vi "FRCts20_Backend_API_Application.vi"(8 "error in (no error)":errorcluster, 10 "Command":T1="Revision") -> (0 "error out":errorcluster, 2 "Status":string, 3 "Application":T2)   [LabVIEW 2014, in "FRCts20_Backend_Engine.lvlib" / "FRCts20_Backend_API.lvlib"]
doc: "This VI could be in charge of controlling the backend, but at present it is not."
uses:
  FRCts20_Backend_API.lvlib
  FRCts20_Backend_API_Application.ctl
  FRCts20_Backend_API_Command_App.ctl
  FRCts20_Backend_FGVOperation.ctl
  FRCts20_Backend_Engine.lvlib
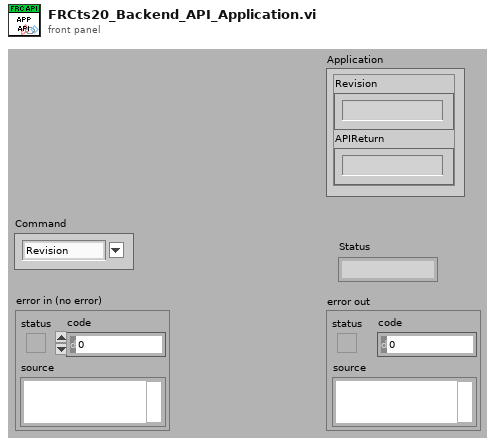
[diagram p1: front panel]
types:
  T1 = typedef "FRCts20_Backend_Engine.lvlib/FRCts20_Backend_API.lvlib/FRCts20_Backend_API_Command_App.ctl" = string
  T2 = typedef "FRCts20_Backend_API_Application.ctl" = cluster{"Revision":string, "APIReturn":string}
  T3 = typedef "FRCts20_Backend_Engine.lvlib/FRCts20_Backend_FGVOperation.ctl" = enum16{"Initialize", "EnqueueMessage", "EnqueueDataReturn", "FlushMessage", "FlushDataReturn"}
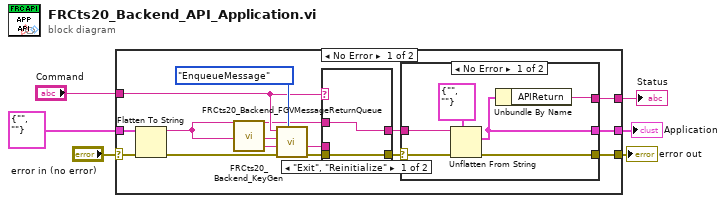
[diagram p0: block diagram]
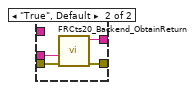
[diagram p2: hidden frame]
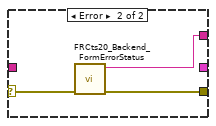
[diagram p3: hidden frame]
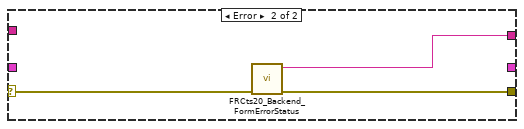
[diagram p4: hidden frame]
diagram:
  n1 = case shown="No Error" "error in (no error)" {
    selector: "error in (no error)" -> [w20 w37]
    tunnel: [w14 w36] -> w5
    tunnel: [w12 w38] -> w4
    tunnel: "Command" -> [w8 _]
    tunnel: [w11 _] -> w2
    tunnel: T2 {"Revision"="", "APIReturn"=""} ("Revision") -> [w10 _]
    frame No Error {
      n2 = Flatten To String(anything=w10, error in (no error)=w20) -> (data string=w7:string, error out=w19:errorcluster)  [unwired: 2 in, 1 out]
      n3 = call "FRCts20_Backend_KeyGen.vi"() -> ("Keygen"=w18:string)  [unwired: 27 in]
      n4 = call "FRCts20_Backend_FGVMessageReturnQueue.vi"("Operation"=FRCts20_Backend_FGVOperation."EnqueueMessage", "error in (no error)"=w19, "Key"=w18, "Message Value"=w7, "Message Name"=w8) -> ("error out"=w16:errorcluster, "Key (Duplicate)"=w15:string)  [unwired: 5 in]
      n5 = case shown="\"Exit\", \"Reinitialize\"" w8 {
        tunnel: w16 -> [w22 w26]
        tunnel: w15 -> [_ w25]
        tunnel: [w22 w24] -> w13
        tunnel: [w21 w23] -> w9
        tunnel: w7 -> [w21 _]
        frame "Exit", "Reinitialize" {
        }
        frame "True", Default {
          n6 = call "FRCts20_Backend_ObtainReturn.vi"("error in (no error)"=w26, "Key"=w25) -> ("error out"=w24:errorcluster, "Message Value"=w23:string)  [unwired: 8 in]
        }
      }
      n7 = case shown="No Error" w13 {
        selector: w13 -> [w31 w35]
        tunnel: [w32 w34] -> w14
        tunnel: [w30 _] -> w11
        tunnel: [w29 w33] -> w12
        tunnel: w9 -> [w27 _]
        frame No Error {
          n8 = Unflatten From String(type=T2 {"Revision"="", "APIReturn"=""} ("Revision"), binary string=w27, error in (no error)=w31) -> (value=w30:T2, error out=w32:errorcluster)  [unwired: 2 in, 1 out]
          n9 = Unbundle By Name(w30) -> ("APIReturn"=w29:string)
        }
        frame Error {
          n10 = call "FRCts20_Backend_FormErrorStatus.vi"("error in (no error)"=w35) -> ("error out"=w34:errorcluster, "String"=w33:string)  [unwired: 9 in]
        }
      }
    }
    frame Error {
      n11 = call "FRCts20_Backend_FormErrorStatus.vi"("error in (no error)"=w37) -> ("error out"=w36:errorcluster, "String"=w38:string)  [unwired: 9 in]
    }
  }
  "error out" <- w5
  "Status" <- w4
  "Application" <- w2
